vi "Get Plugin Metadata.vi"(8 "error in (no error)":errorcluster, 11 "Packed Library Path":path) -> (0 "error out":errorcluster, 3 "Plugin Metadata":T1)   [LabVIEW 2021, in "CIFLauncher.lvclass"]
uses:
  CIFLauncher.lvclass
  CIFLauncher.lvclass/CIFLauncher.ctl
  <vilib>/Utility/LVLibp/NI_PackedLibraryUtility.lvlib
  typedef/trash_Plugin Metadata.ctl
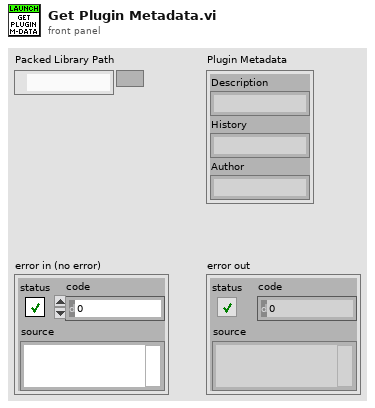
[diagram p1: front panel]
types:
  T1 = typedef "trash_Plugin Metadata.ctl" = cluster{"Description":string, "History":string, "Author":string}
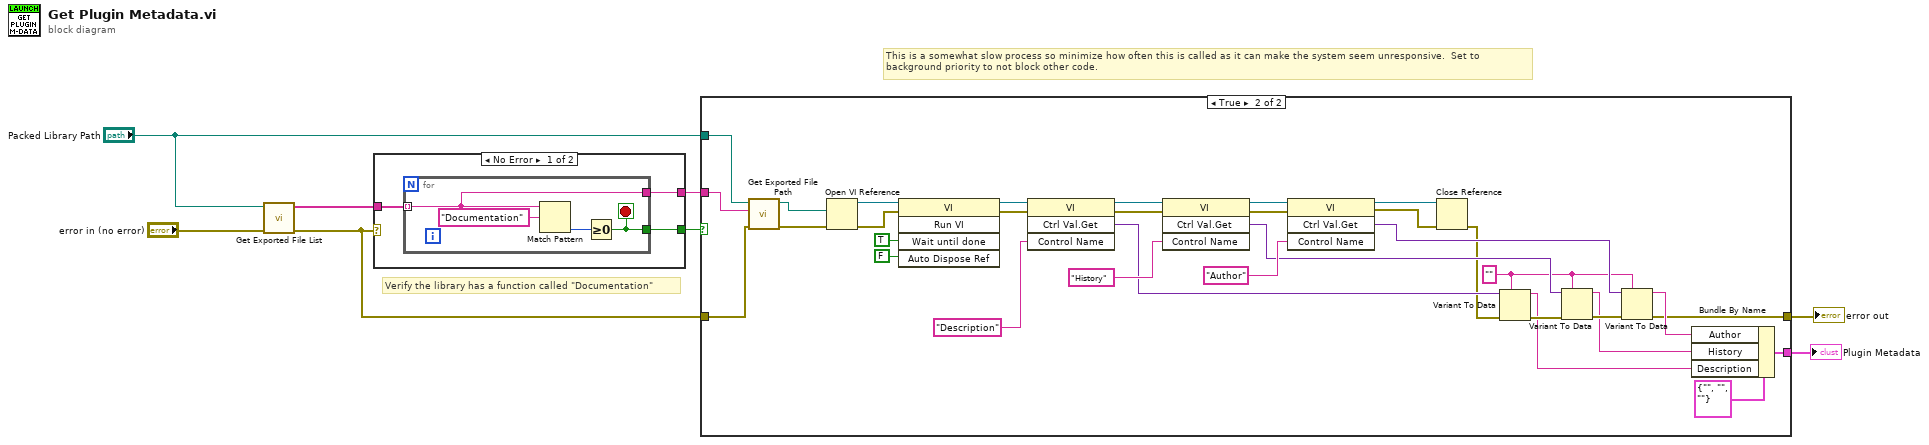
[diagram p0: block diagram]
diagram:
  # "This is a somewhat slow process so minimize how often this is called as it can make the system seem unresponsive.  Set to background priority to not block other code."
  # "Verify the library has a function called \"Documentation\""
  n1 = call <vilib>:"Get Exported File List.vi"("error in (no error)"="error in (no error)", "packed library path"="Packed Library Path") -> ("error out"=w2:errorcluster, "qualified names"=w6:string[])  [unwired: 7 in, 1 out]
  n2 = case shown="No Error" w2 {
    tunnel: w6 -> [w11 _]
    tunnel: [w10 _] -> w3
    tunnel: [w9 _] -> w5
    frame No Error {
      n3 = for {
        tunnel: w11 -> [w13] mode=indexing
        tunnel: [w14] -> w10
        tunnel: [w13] -> w9
        stop <- w14 stop-if-true
        n4 = Match Pattern(string=w13, regular expression="Documentation") -> (offset past match=w15:i32)  [unwired: 1 in, 3 out]
        n5 = Greater Or Equal To 0?(x=w15) -> (x >= 0?=w14:bool)
      }
    }
    frame Error {
    }
  }
  n6 = case shown="True" w3 {
    tunnel: [w16 w22] -> w8
    tunnel: [_ w49] -> w7
    tunnel: w5 -> [_ w47]
    tunnel: "Packed Library Path" -> [_ w24]
    tunnel: w2 -> [w16 w23]
    frame False {
    }
    frame True {
      w29 = "" ("Control Name")
      n7 = call <vilib>:"Get Exported File Path.vi"("error in (no error)"=w23, "qualified name"=w47, "packed library path"=w24) -> ("error out"=w19:errorcluster, "path"=w48:path)  [unwired: 7 in]
      n8 = Open VI Reference(vi path=w48, error in (no error)=w19) -> (vi reference=w46:refnum<vi>, error out=w20:errorcluster)  [unwired: 4 in]
      n9 = invoke class="VI" method="Run VI"(reference=w46, error in=w20, "Wait until done"=TRUE ("Wait Until Done"), "Auto Dispose Ref"=FALSE ("Auto Dispose Reference")) -> (reference out=w45:refnum<vi>, error out=w21:errorcluster)  [unwired: 1 in, 3 out]
      n10 = invoke class="VI" method="Ctrl Val.Get"(reference=w45, error in=w21, "Control Name"="Description") -> (reference out=w43:refnum<vi>, error out=w42:errorcluster, "Get Control Value Variant"=w32:variant)  [unwired: 1 in, 1 out]
      n11 = invoke class="VI" method="Ctrl Val.Get"(reference=w43, error in=w42, "Control Name"="History") -> (reference out=w39:refnum<vi>, error out=w38:errorcluster, "Get Control Value Variant"=w31:variant)  [unwired: 1 in, 1 out]
      n12 = invoke class="VI" method="Ctrl Val.Get"(reference=w39, error in=w38, "Control Name"="Author") -> (reference out=w37:refnum<vi>, error out=w36:errorcluster, "Get Control Value Variant"=w33:variant)  [unwired: 1 in, 1 out]
      n13 = Close Reference(reference=w37, error in (no error)=w36) -> (error out=w30:errorcluster)
      n14 = Variant To Data(error in=w30, type=w29, Variant=w32) -> (data=w26:string, error out=w35:errorcluster)
      n15 = Variant To Data(error in=w35, type=w29, Variant=w31) -> (data=w25:string, error out=w34:errorcluster)
      n16 = Variant To Data(error in=w34, type=w29, Variant=w33) -> (data=w27:string, error out=w22:errorcluster)
      n17 = Bundle By Name(cluster=T1 {"Description"="", "History"="", "Author"=""} ("Plugin Metadata"), "Author"=w27, "History"=w25, "Description"=w26) -> (w49:T1)
    }
  }
  "error out" <- w8
  "Plugin Metadata" <- w7
